vi "SGL_to_4_byte_array.vi"(0 "SGL float":sgl format="%.2f") -> (1 "SGL float encoded array of bytes":u8[](array[numeric]), 2 "bytes":u32)   [LabVIEW 2017]
doc: "Convert a SGL precision float to an array of 4 bytes.\nConversion according to IEEE 754-1990.\n\nThis VI is used together with the VI AMB_Control which requires all parameters to be sent as bytes."
panel:
  # "Convert DBL float to array of 8 bytes IEEE 754-1990 \nC.Holmstedt 2002-03-06"
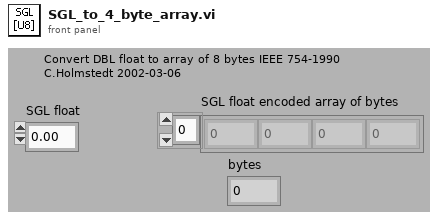
[diagram p1: front panel]
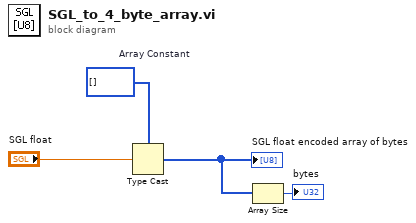
[diagram p0: block diagram]
diagram:
  w1 = u8[] []  # Array Constant
  n1 = Type Cast(type=w1, x="SGL float") -> (*(type *) &x=w3:u8[])
  "SGL float encoded array of bytes" <- w3
  n2 = Array Size(array=w3) -> (size(s)=→"bytes":i32)
